vi "Rapid Filter Tester.vi"() -> ()   [LabVIEW 2012]
doc: "Changed serial pause logic for sending commands to the STAMP box to ensure that it can never be less than the minimum value.\n\nIncreased serial pause from 50 to 75 ms."
uses:
  file action.ctl
  Pump calibration/calibration commands.ctl
  Sample commands.ctl
  sample references.ctl
  Peristaltic/3-stop colors.ctl
  State Setting.ctl
  tanks.ctl
  tank.ctl
  Method settings.ctl
  column flow.ctl
  point.ctl
  vial position.ctl
  sampler states.ctl
  sample array.ctl
  legend.ctl
  toolbar icons/help.ctl
  Peristaltic/Pump.ctl
  mini peristaltic pump.ctl
  Pump Direction.ctl
  RACE  compact controls.ctl
  Stamp/Switch settings vertical.ctl
  flow fraction.ctl
panel:
  in  "Tab Control":enum32{"Method", "States", "Samples", "Run"}(tab)
  in  "Method settings":T1 {"Column"."porosity" format="%.4f"; "Column"."diameter" format="%.2f"; "Column"."length" format="%.2f"}
  in  "Test list":i32(listbox)
  in  "add cycle before":bool
  in  "delete cycle":bool
  in  "Test name":string="first cycle"
  in  "add cycle after":bool
  in  "State Settings":T3[][](array[typedef])=[[{"switches"={"Pump"=FALSE, "1"=FALSE, "2"=FALSE, "3"=FALSE, "4"=FALSE, "5"=FALSE, "6"=FALSE}, "flow rate"=0.0, "flow division"={"1"=0.0, "2"=0.0, "3"=0.0, "4"=0.0, "5"=0.0}, "State name"="", "state duration"=0.0, "valve cycle time"=0.2}]] {"valve cycle time" min=0.2 step=0.1 format="%.2f"; "flow division"."5" min=0.0 max=1.0 step=0.01 format="%.3f"; "flow division"."4" min=0.0 max=1.0 step=0.01 format="%.3f"; "flow division"."3" min=0.0 max=1.0 step=0.01 format="%.3f"; "flow division"."2" min=0.0 max=1.0 step=0.01 format="%.3f"; "flow division"."1" min=0.0 max=1.0 step=0.01 format="%.3f"; "flow rate" format="%.3f"}
  in  "Influent list":i32(listbox)
  in  "add state before":bool
  in  "delete state":bool
  in  "State name":string="first reagent"
  in  "add state after":bool
  out "Legend":T6
  in  "Sample array":T7 {"Sample volume" format="%.2f"; "Influent list" items=["first reagent"]; "Test list" items=["first cycle"]; "t/theta" min=0.0 step=0.1}
  in  "Index":i32
  in  "Plant Mode of Operation":T8(ring)=enum."Automatic Operation"
  in  "stop run":bool
  in  "Run":bool
  out "valve cycle time":dbl[unit] format="%.2f"
  in  "Help Button":T9
  in  "Calibrate Pump":T10 {"flow rate" format="%.2f"}
  out "Sample Tray":T12
  out "Sample plot":picture
  out "sampler state":T13
  out "vial position":T14
  out "run done":bool
  out "current time":dbl[unit]
  out "column flow":T15 {"t/q" format="%.3f"; "Velocity" format="%.3f"}
  in  "Which volumes":T16(ring)
  out "total run time":dbl[unit]
  out "update gui":bool=TRUE
  out "Elapsed time in current state":dbl[unit] format="%<%H:%M:%S%2u>t"
  in  "Reagents":string[](array[string])
  in  "New State":T3={"switches"={"Pump"=FALSE, "1"=FALSE, "2"=FALSE, "3"=FALSE, "4"=FALSE, "5"=FALSE, "6"=FALSE}, "flow rate"=0.0, "flow division"={"1"=0.0, "2"=0.0, "3"=0.0, "4"=0.0, "5"=0.0}, "State name"="", "state duration"=0.0, "valve cycle time"=0.2} {"valve cycle time" min=0.2 step=0.1 format="%.2f"; "flow division"."5" min=0.0 max=1.0 step=0.01 format="%.3f"; "flow division"."4" min=0.0 max=1.0 step=0.01 format="%.3f"; "flow division"."3" min=0.0 max=1.0 step=0.01 format="%.3f"; "flow division"."2" min=0.0 max=1.0 step=0.01 format="%.3f"; "flow division"."1" min=0.0 max=1.0 step=0.01 format="%.3f"; "flow rate" format="%.3f"}
  out "Quit":bool
  out "Control Settings":T17
  out "tanks":T20 {"Tank 5" scale format="%.1f"; "Tank 4" scale format="%.1f"; "Tank 3" scale format="%.1f"; "Tank 2" scale format="%.1f"; "Tank 1" scale format="%.1f"}
  # "sampler"
  # "waste"
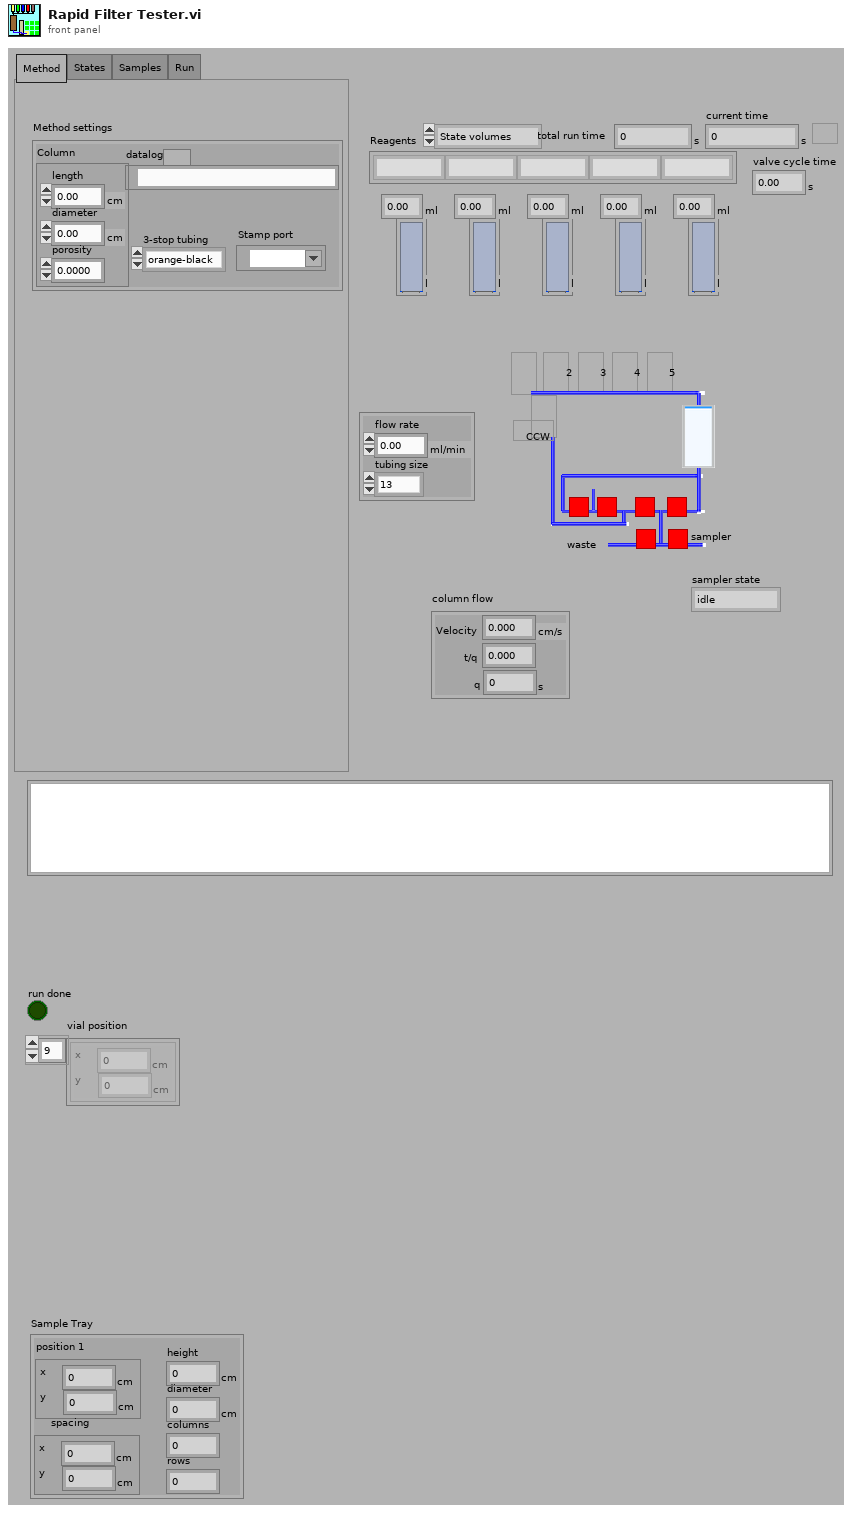
[diagram p1: front panel]
types:
  T1 = typedef "Method settings.ctl" = cluster{"3-stop tubing":T2, "Stamp port":refnum<visa-resource-name>, "datalog":path, "Column":cluster{"length":dbl[unit], "diameter":dbl[unit], "porosity":dbl}}
  T2 = typedef "3-stop colors.ctl" = enum16{"orange-black", "orange-red", "orange-blue", "orange-green", "green-yellow", "orange-yellow", "white-yellow", "orange-white", "black-black", "orange-orange", "white-black", "white-white", "white-red", "red-red", "red-grey", "grey-grey", "yellow-yellow", "yellow-blue", "blue-blue", "blue-green", "green-green", "purple-purple", "purple-black", "purple-orange", "purple-white", "black-white", "13", "14", "15", "16", "17", "18"}
  T3 = typedef "State Setting.ctl" = cluster{"switches":T4, "flow rate":dbl[unit], "flow division":cluster{"1":T5, "2":T5, "3":T5, "4":T5, "5":T5}, "State name":string, "state duration":dbl[unit], "valve cycle time":dbl[unit]}
  T4 = typedef "Switch settings vertical.ctl" = cluster{"Pump":bool, "1":bool, "2":bool, "3":bool, "4":bool, "5":bool, "6":bool}
  T5 = typedef "flow fraction.ctl" = dbl
  T6 = typedef "legend.ctl" = cluster{"Feed ":string, "Color":u32}[]
  T7 = typedef "sample array.ctl" = cluster{"start time":dbl[unit], "end time":dbl[unit], "t/theta":dbl, "Test list":u16, "Influent list":u16, "Sample volume":dbl[unit], "Too close to previous sample":bool}[]
  T8 = enum16{"Operator Selected State", "Automatic Operation"}
  T9 = typedef "help.ctl" = bool
  T10 = typedef "Pump.ctl" = cluster{"tubing size":enum16{"13", "14", "16", "25", "17", "18"}, "flow rate":dbl[unit]}
  T11 = typedef "point.ctl" = cluster{"x":dbl[unit], "y":dbl[unit]}
  T12 = cluster{"diameter":dbl[unit], "height":dbl[unit], "columns":u16, "rows":u16, "position 1":T11, "spacing":T11}
  T13 = typedef "sampler states.ctl" = enum16{"idle", "go sample loc", "collect sample", "go home"}
  T14 = typedef "vial position.ctl" = T11[]
  T15 = typedef "column flow.ctl" = cluster{"Velocity":dbl[unit], "t/q":dbl, "q":dbl[unit]}
  T16 = enum16{"State volumes", "Cycle volumes", "Experiment volumes"}
  T17 = typedef "RACE  compact controls.ctl" = cluster{"Switches":cluster{"1":T18, "2":T18, "3":T18, "4":T18, "5":T18, "Boolean":bool, "Boolean 2":bool, "Boolean 3":bool, "Boolean 4":bool, "Boolean 5":bool, "Boolean 6":bool, "main pump":T18, "direction":T19}}
  T18 = typedef "mini peristaltic pump.ctl" = bool
  T19 = typedef "Pump Direction.ctl" = bool
  T20 = typedef "tanks.ctl" = cluster{"Tank 1":T21, "Tank 2":T21, "Tank 3":T21, "Tank 4":T21, "Tank 5":T21}
  T21 = typedef "tank.ctl" = dbl[unit]
  T22 = typedef "calibration commands.ctl" = enum16{"Get ini Path", "Save default values", "Save new calibration", "Read calibration", "Apply calibration", "Read STAMP mb", "Write STAMP mb"}
  T23 = typedef "sample references.ctl" = cluster{"Index":refnum<vi>, "Test list":refnum<vi>, "Influent list":refnum<vi>, " State Settings":refnum<vi>, "Method settings":refnum<vi>, "Sample plot":refnum<vi>, "Legend":refnum<vi>, "Test Ring":refnum<vi>, "Influent Ring":refnum<vi>, "TabCtl Refnum":refnum<vi>, "Sample array":refnum<vi>}
  T24 = typedef "Sample commands.ctl" = enum16{"Configure", "Update times", "Index", "Update rings", "Plot current time"}
  T25 = typedef "file action.ctl" = enum16{"Save", "Open"}
  T26 = typedef "calibration values.ctl" = cluster{"target 1":dbl[unit], "target 2":dbl[unit], "measured 1":dbl[unit], "measured 2":dbl[unit]}
  T27 = typedef "Stamp Controls.ctl" = cluster{"Pump speed":dbl, "switches":T28}
  T28 = typedef "switches.ctl" = cluster{"Pump":bool, "1":bool, "2":bool, "3":bool, "4":bool, "5":bool, "6":bool}
  T29 = cluster{"Item Names":string[], "Value":i32, "Item Names":string[], "Value":i32, " State Settings":T3[][], "Method settings":T1, "Reagents":string[], "vial position":T14, "Sample array":T7, "Sample Tray":cluster{"diameter":dbl[unit], "height":dbl[unit], "columns":u16, "rows":u16, "position 1":T11, "spacing":T11}}
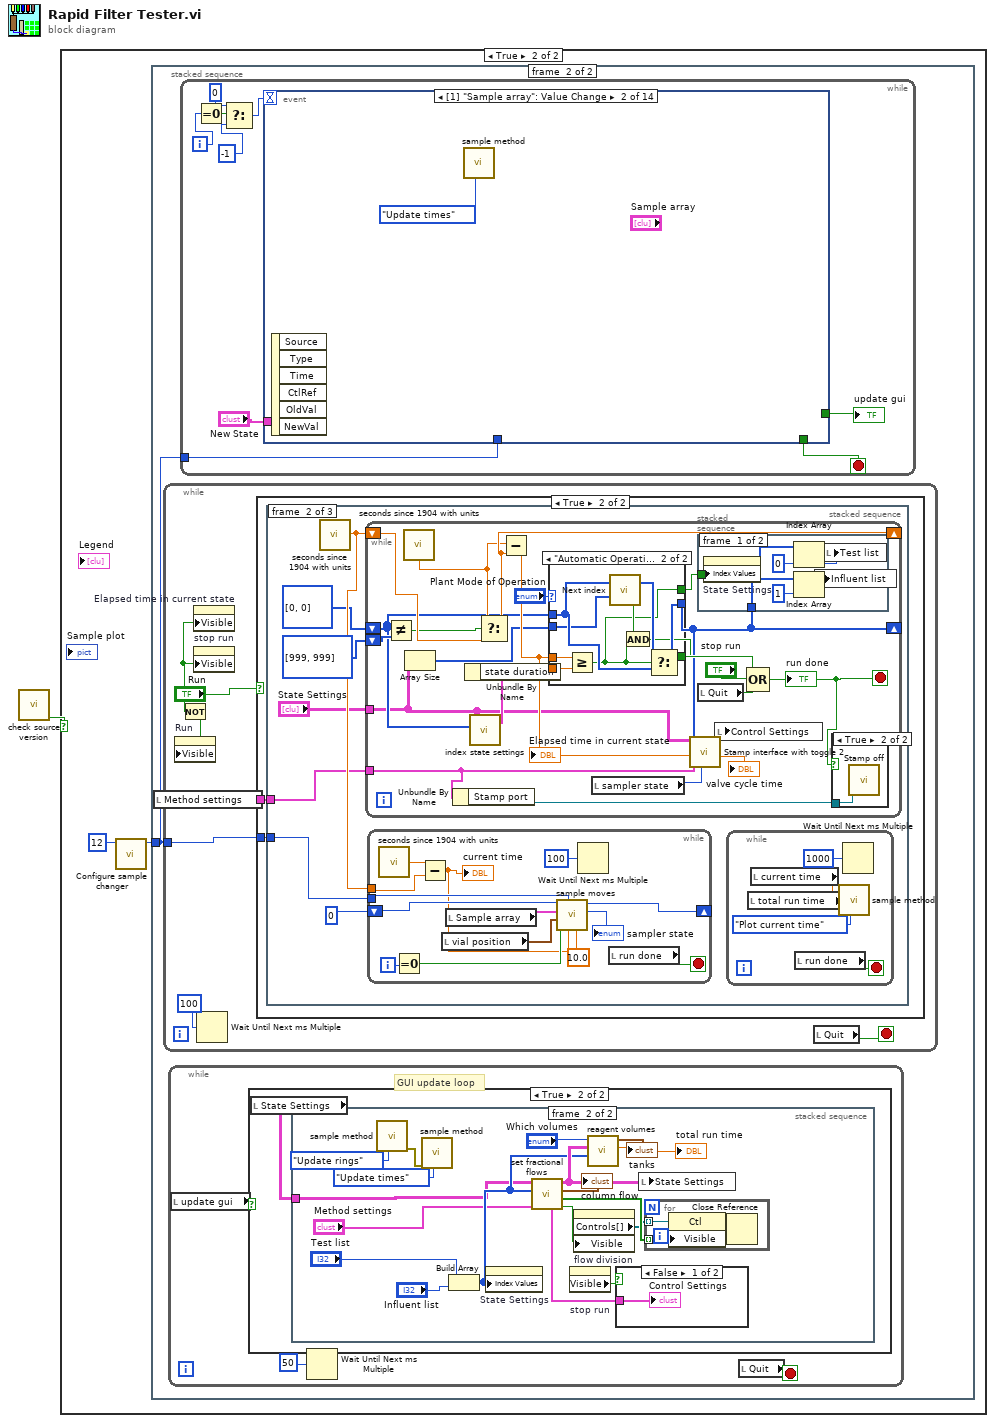
[diagram p0: block diagram]
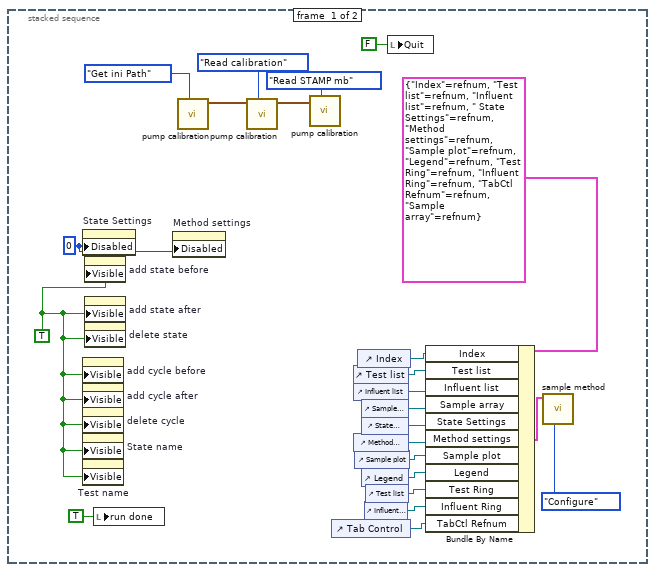
[diagram p3: hidden frame]
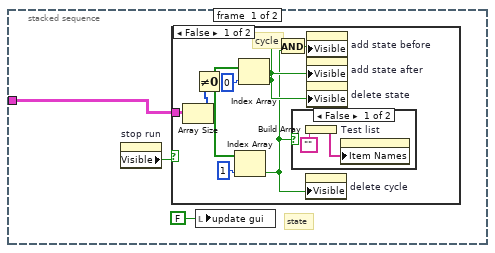
[diagram p5: hidden frame]
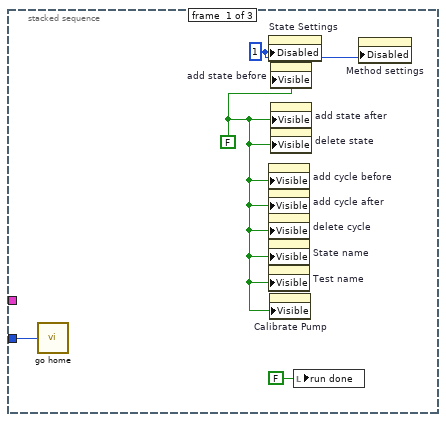
[diagram p10: hidden frame]
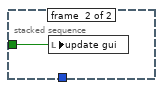
[diagram p12: hidden frame]
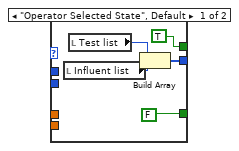
[diagram p13: hidden frame]
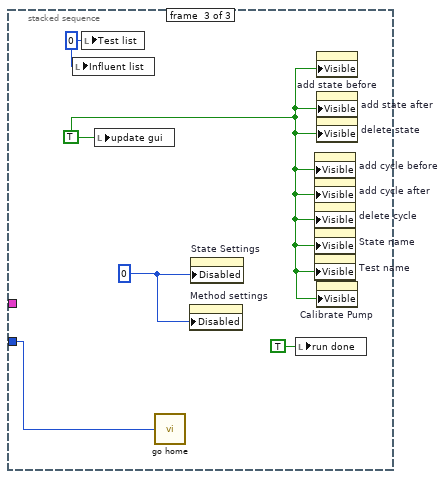
[diagram p14: hidden frame]
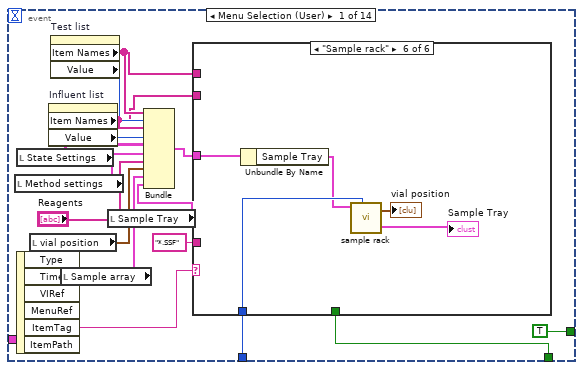
[diagram p15: hidden frame]
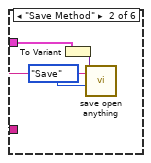
[diagram p17: hidden frame]
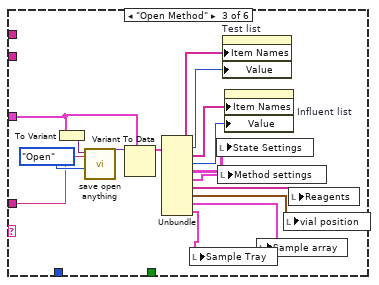
[diagram p18: hidden frame]
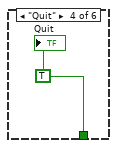
[diagram p19: hidden frame]
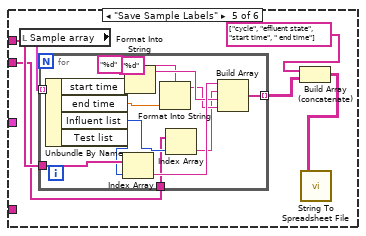
[diagram p20: hidden frame]
diagram:
  n1 = call "check source version.vi"() -> ("continue running?"=w1:bool)  [unwired: 2 in, 3 out]
  n2 = case shown="True" w1 {
    frame False {
    }
    frame True {
      n3 = call "Configure sample changer.vi"("ID"=12) -> ("ID out"=w2:i32)  [unwired: 6 in]
      n4 = stacked-sequence {
        tunnel: w2 -> [_ w27]
        frame #0 {
          w24 = u8 0 ("Disabled")
          w25 = TRUE
          n5 = property on="State Settings" class="Arr (strict)"("Disabled"=w24) -> ()  [unwired: 2 in, 2 out]
          n6 = property on="add cycle before" class="Bool"("Visible"=w25) -> ()  [unwired: 2 in, 2 out]
          n7 = property on="add cycle after" class="Bool"("Visible"=w25) -> ()  [unwired: 2 in, 2 out]
          n8 = property on="delete cycle" class="Bool"("Visible"=w25) -> ()  [unwired: 2 in, 2 out]
          n9 = property on="State name" class="Str"("Visible"=w25) -> ()  [unwired: 2 in, 2 out]
          n10 = property on="Test name" class="Str"("Visible"=w25) -> ()  [unwired: 2 in, 2 out]
          n11 = property on="add state before" class="Bool"("Visible"=w25) -> ()  [unwired: 2 in, 2 out]
          n12 = property on="add state after" class="Bool"("Visible"=w25) -> ()  [unwired: 2 in, 2 out]
          n13 = property on="delete state" class="Bool"("Visible"=w25) -> ()  [unwired: 2 in, 2 out]
          n14 = local write "run done"(TRUE ("run done")) -> ()
          n15 = property on="Method settings" class="Clust (strict)"("Disabled"=w24) -> ()  [unwired: 2 in, 2 out]
          n16 = call "pump calibration.vi"("pump cal command"=calibration_commands."Get ini Path") -> ("Pump Calibration out"=w21:T26)  [unwired: 4 in, 3 out]
          n17 = call "pump calibration.vi"("pump cal command"=calibration_commands."Read calibration", "Pump Calibration in"=w21) -> ("Pump Calibration out"=w5:T26)  [unwired: 3 in, 3 out]
          n18 = call "pump calibration.vi"("pump cal command"=calibration_commands."Read STAMP mb", "Pump Calibration in"=w5) -> ()  [unwired: 3 in, 4 out]
          n19 = control-ref of="Tab Control"() -> (w7:refnum<vi>)
          n20 = control-ref of="Test list"() -> (w16:refnum<vi>)
          n21 = control-ref of="Influent list"() -> (w15:refnum<vi>)
          n22 = control-ref of="Method settings"() -> (w12:refnum<vi>)
          n23 = control-ref of="Sample plot"() -> (w11:refnum<vi>)
          n24 = control-ref of="Index"() -> (w17:refnum<vi>)
          n25 = control-ref of="Sample array"() -> (w14:refnum<vi>)
          n26 = control-ref of="State Settings"() -> (w13:refnum<vi>)
          n27 = control-ref of="Legend"() -> (w10:refnum<vi>)
          n28 = control-ref of="Influent list"() -> (w8:refnum<vi>)
          n29 = control-ref of="Test list"() -> (w9:refnum<vi>)
          n30 = local write "Quit"(FALSE ("Quit")) -> ()
          n31 = Bundle By Name(cluster=T23 {"Index"=refnum, "Test list"=refnum, "Influent list"=refnum, " State Settings"=refnum, "Method settings"=refnum, "Sample plot"=refnum, "Legend"=refnum, "Test Ring"=refnum, "Influent Ring"=refnum, "TabCtl Refnum"=refnum, "Sample array"=refnum} ("Ref cluster"), "Index"=w17, "Test list"=w16, "Influent list"=w15, "Sample array"=w14, "State Settings"=w13, "Method settings"=w12, "Sample plot"=w11, "Legend"=w10, "Test Ring"=w9, "Influent Ring"=w8, "TabCtl Refnum"=w7) -> (w18:T23)
          n32 = call "sample method.vi"("Sample Commands"=Sample_commands."Configure", "Ref cluster"=w18) -> ()  [unwired: 9 in, 1 out]
        }
        frame #1 {
          n33 = while {
            tunnel: w27 -> [w69]
            stop <- w71 stop-if-true
            n34 = local read "Method settings"() -> (w68:T1)
            n35 = Not(x="Run") -> (.not. x?=w72:bool)
            n36 = property on="Run" class="Bool"("Visible"=w72) -> ()  [unwired: 2 in, 2 out]
            n37 = property on="Elapsed time in current state" class="DigNum (strict)"("Visible"="Run") -> ()  [unwired: 2 in, 2 out]
            n38 = property on="stop run" class="Bool"("Visible"="Run") -> ()  [unwired: 2 in, 2 out]
            n39 = Wait Until Next ms Multiple(millisecond multiple=u32 100) -> ()  [unwired: 1 out]
            n40 = case shown="True" "Run" {
              tunnel: w69 -> [_ w74]
              tunnel: w68 -> [_ w73]
              frame False {
              }
              frame True {
                n41 = stacked-sequence {
                  tunnel: w74 -> [w76 w82 w150]
                  tunnel: w73 -> [_ w79 _]
                  frame #0 {
                    w77 = u8 1 ("Disabled")
                    w75 = FALSE
                    n42 = call "go home.vi"("ID in"=w76) -> ()
                    n43 = property on="State Settings" class="Arr (strict)"("Disabled"=w77) -> ()  [unwired: 2 in, 2 out]
                    n44 = property on="add cycle before" class="Bool"("Visible"=w75) -> ()  [unwired: 2 in, 2 out]
                    n45 = property on="add cycle after" class="Bool"("Visible"=w75) -> ()  [unwired: 2 in, 2 out]
                    n46 = property on="delete cycle" class="Bool"("Visible"=w75) -> ()  [unwired: 2 in, 2 out]
                    n47 = property on="State name" class="Str"("Visible"=w75) -> ()  [unwired: 2 in, 2 out]
                    n48 = property on="Test name" class="Str"("Visible"=w75) -> ()  [unwired: 2 in, 2 out]
                    n49 = property on="Calibrate Pump" class="Clust (strict)"("Visible"=w75) -> ()  [unwired: 2 in, 2 out]
                    n50 = property on="add state before" class="Bool"("Visible"=w75) -> ()  [unwired: 2 in, 2 out]
                    n51 = property on="add state after" class="Bool"("Visible"=w75) -> ()  [unwired: 2 in, 2 out]
                    n52 = property on="delete state" class="Bool"("Visible"=w75) -> ()  [unwired: 2 in, 2 out]
                    n53 = local write "run done"(FALSE ("run done")) -> ()
                    n54 = property on="Method settings" class="Clust (strict)"("Disabled"=w77) -> ()  [unwired: 2 in, 2 out]
                  }
                  frame #1 {
                    n55 = call "seconds since 1904 with units.vi"() -> ("seconds since 1Jan1904"=w84:dbl[unit])
                    n56 = while {
                      shift-right: [w115] -> _
                      shift-left: u32[] [999, 999] ("Index Values") -> [w122]
                      shift-left: u32[] [0, 0] ("Index Values") -> [w109]
                      shift-right: [w125] -> _
                      shift-left: w84 -> [w126]
                      tunnel: "State Settings" -> [w108]
                      tunnel: w79 -> [w106]
                      stop <- w105 stop-if-true
                      n57 = Not Equal?(x=w109, y=w122) -> (x != y?=w114:bool)
                      n58 = call "seconds since 1904 with units.vi"() -> ("seconds since 1Jan1904"=w112:dbl[unit])
                      n59 = Array Size(array=w108) -> (size(s)=w116:i32[])
                      n60 = Unbundle By Name(w106) -> ("Stamp port"=w107:refnum<visa-resource-name>)
                      n61 = call "index state settings.vi"("Next Index"=w109, "State Settings"=w108) -> ("State"=w118:T3)  [unwired: 2 in, 1 out]
                      n62 = Unbundle By Name(w118) -> ("state duration"=w124:dbl[unit])
                      n63 = Select(t=w112, s=w114, f=w126) -> (s? t:f=w125:dbl[unit])
                      n64 = Subtract(x=w112, y=w125) -> (x-y=w123:dbl[unit])
                      "Elapsed time in current state" <- w123
                      n65 = case shown="\"Automatic Operation\"" "Plant Mode of Operation" {
                        tunnel: [w137 w145] -> w115
                        tunnel: w123 -> [_ w148]
                        tunnel: w124 -> [_ w147]
                        tunnel: w109 -> [_ w144]
                        tunnel: [FALSE ("last state") w141] -> w119
                        tunnel: w116 -> [_ w143]
                        tunnel: [TRUE w140] -> w113
                        frame "Operator Selected State", Default {
                          n66 = local read "Influent list"() -> (w138:i32)
                          n67 = local read "Test list"() -> (w139:i32)
                          n68 = Build Array(w139, w138) -> (w137:i32[])
                        }
                        frame "Automatic Operation" {
                          n69 = Greater Or Equal?(x=w148, y=w147) -> (x >= y?=w140:bool)
                          n70 = call "Next index.vi"("size(s)"=w143, "Current Index"=w144) -> ("last state"=w142:bool, "Next Index"=w146:u32[])
                          n71 = And(x=w142, y=w140) -> (x .and. y?=w141:bool)
                          n72 = Select(t=w146, s=w140, f=w144) -> (s? t:f=w145:u32[])
                        }
                      }
                      n73 = local read "sampler state"() -> (w111:T13)
                      n74 = call "Stamp interface with toggle 2.vi"("sampler state"=w111, "Elapsed time in current state"=w123, "Method settings"=w106, "Index"=w115, "State Settings"=w108) -> ("valve cycle time"=→"valve cycle time":dbl[unit], "Controls out"=w117:T27)  [unwired: 4 in, 1 out]
                      n75 = stacked-sequence {
                        tunnel: w115 -> [w132 _]
                        tunnel: w113 -> [_ w134]
                        frame #0 {
                          n76 = property on="State Settings" class="Arr (strict)"("Index Values"=w132) -> ()  [unwired: 2 in, 2 out]
                          n77 = Index Array(array=w132, index=0) -> (element=w133:u32)
                          n78 = Index Array(array=w132, index=1) -> (element=w131:u32)
                          n79 = local write "Influent list"(w131) -> ()
                          n80 = local write "Test list"(w133) -> ()
                        }
                        frame #1 {
                          n81 = local write "update gui"(w134) -> ()
                        }
                      }
                      n82 = local read "Quit"() -> (w120:bool)
                      n83 = local write "Control Settings"(w117) -> ()
                      n84 = Compound Arithmetic op=OR(w119, "stop run", w120) -> (w105:bool)
                      "run done" <- w105
                      n85 = case shown="True" w105 {
                        tunnel: w107 -> [_ w128]
                        frame False {
                        }
                        frame True {
                          n86 = call "Stamp off.vi"("Serial Port"=w128) -> ()  [unwired: 9 in, 2 out]
                        }
                      }
                    }
                    n87 = while {
                      tunnel: w84 -> [w102]
                      shift-right: [w100] -> _
                      shift-left: 0 -> [w101]
                      tunnel: w82 -> [w97]
                      i -> [w93]
                      stop <- w104 stop-if-true
                      n88 = call "seconds since 1904 with units.vi"() -> ("seconds since 1Jan1904"=w103:dbl[unit])
                      n89 = Equal To 0?(x=w93) -> (x = 0?=w92:bool)
                      n90 = Subtract(x=w103, y=w102) -> (x-y=w91:dbl[unit])
                      "current time" <- w91
                      n91 = local read "vial position"() -> (w94:T14)
                      n92 = local read "Sample array"() -> (w98:T7)
                      n93 = call "sample moves.vi"("move time"=dbl[unit] 10.0, "current time"=w91, "Gilson ID"=w97, "initialize"=w92, "vial position"=w94, "Samples"=w98, "sample ID"=w101) -> ("sampler state"=→"sampler state":T13, "sample ID out"=w100:i16)  [unwired: 3 in]
                      n94 = Wait Until Next ms Multiple(millisecond multiple=u32 100) -> ()  [unwired: 1 out]
                      n95 = local read "run done"() -> (w104:bool)
                    }
                    n96 = while {
                      stop <- w90 stop-if-true
                      n97 = local read "total run time"() -> (w88:dbl[unit])
                      n98 = local read "current time"() -> (w87:dbl[unit])
                      n99 = local read "run done"() -> (w90:bool)
                      n100 = call "sample method.vi"("Sample Commands"=Sample_commands."Plot current time", "total run time"=w88, "current time"=w87) -> ()  [unwired: 8 in, 1 out]
                      n101 = Wait Until Next ms Multiple(millisecond multiple=u32 1000) -> ()  [unwired: 1 out]
                    }
                  }
                  frame #2 {
                    w151 = u8 0 ("Disabled")
                    w153 = 0 ("Cycle list")
                    w149 = TRUE ("update gui")
                    n102 = local write "Influent list"(w153) -> ()
                    n103 = local write "Test list"(w153) -> ()
                    n104 = local write "update gui"(w149) -> ()
                    n105 = call "go home.vi"("ID in"=w150) -> ()
                    n106 = property on="Method settings" class="Clust (strict)"("Disabled"=w151) -> ()  [unwired: 2 in, 2 out]
                    n107 = property on="State Settings" class="Arr (strict)"("Disabled"=w151) -> ()  [unwired: 2 in, 2 out]
                    n108 = local write "run done"(TRUE ("run done")) -> ()
                    n109 = property on="add cycle before" class="Bool"("Visible"=w149) -> ()  [unwired: 2 in, 2 out]
                    n110 = property on="add cycle after" class="Bool"("Visible"=w149) -> ()  [unwired: 2 in, 2 out]
                    n111 = property on="delete cycle" class="Bool"("Visible"=w149) -> ()  [unwired: 2 in, 2 out]
                    n112 = property on="State name" class="Str"("Visible"=w149) -> ()  [unwired: 2 in, 2 out]
                    n113 = property on="Test name" class="Str"("Visible"=w149) -> ()  [unwired: 2 in, 2 out]
                    n114 = property on="add state before" class="Bool"("Visible"=w149) -> ()  [unwired: 2 in, 2 out]
                    n115 = property on="add state after" class="Bool"("Visible"=w149) -> ()  [unwired: 2 in, 2 out]
                    n116 = property on="delete state" class="Bool"("Visible"=w149) -> ()  [unwired: 2 in, 2 out]
                    n117 = property on="Calibrate Pump" class="Clust (strict)"("Visible"=w149) -> ()  [unwired: 2 in, 2 out]
                  }
                }
              }
            }
            n118 = local read "Quit"() -> (w71:bool)
          }
          n119 = while {
            stop <- w29 stop-if-true
            # "GUI update loop"
            n120 = local read "update gui"() -> (w28:bool)
            n121 = case shown="True" w28 {
              frame False {
              }
              frame True {
                n122 = local read "State Settings"() -> (w31:T3[][])
                n123 = stacked-sequence {
                  tunnel: w31 -> [w34 w48]
                  frame #0 {
                    # "state"
                    n124 = property on="stop run" class="Bool"() -> ("Visible"=w32:bool)  [unwired: 2 in, 2 out]
                    n125 = case shown="False" w32 {
                      tunnel: w34 -> [w36 _]
                      frame False {
                        # "cycle"
                        n126 = Array Size(array=w36) -> (size(s)=w39:i32[])
                        n127 = Not Equal To 0?(x=w39) -> (x != 0?=w40:bool[])
                        n128 = Index Array(array=w40, index=1) -> (element=w35:bool)
                        n129 = Index Array(array=w40, index=0) -> (element=w41:bool)
                        n130 = And(x=w41, y=w35) -> (x .and. y?=w42:bool)
                        n131 = case shown="False" w35 {
                          frame False {
                            n132 = Build Array("") -> (w43:string[])
                            n133 = property on="Test list" class="LstBox (strict)"("Item Names"=w43) -> ()  [unwired: 2 in, 2 out]
                          }
                          frame True {
                          }
                        }
                        n134 = property on="delete cycle" class="Bool"("Visible"=w35) -> ()  [unwired: 2 in, 2 out]
                        n135 = property on="add state before" class="Bool"("Visible"=w42) -> ()  [unwired: 2 in, 2 out]
                        n136 = property on="add state after" class="Bool"("Visible"=w41) -> ()  [unwired: 2 in, 2 out]
                        n137 = property on="delete state" class="Bool"("Visible"=w41) -> ()  [unwired: 2 in, 2 out]
                      }
                      frame True {
                      }
                    }
                    n138 = local write "update gui"(FALSE ("update gui")) -> ()
                  }
                  frame #1 {
                    n139 = call "sample method.vi"("Sample Commands"=Sample_commands."Update rings") -> ("error out"=w45:errorcluster)  [unwired: 10 in]
                    n140 = call "sample method.vi"("Sample Commands"=Sample_commands."Update times", "error in (no error)"=w45) -> ()  [unwired: 9 in, 1 out]
                    n141 = Build Array("Test list", "Influent list") -> (w54:i32[])
                    n142 = property on="State Settings" class="Arr (strict)"("Index Values"=w54) -> ()  [unwired: 2 in, 2 out]
                    n143 = call "set fractional flows.vi"("State Settings"=w48, "Index Values"=w54, "Method settings"="Method settings") -> ("Control Settings"=w60:T27, "State Settings out"=w61:T3[][], "column flow"=→"column flow":T15, "toggle valves"=w58:bool[], "show fractions"=w59:bool)  [unwired: 2 in]
                    n144 = property on="stop run" class="Bool"() -> ("Visible"=w56:bool)  [unwired: 2 in, 2 out]
                    n145 = property on="flow division" class="Clust (strict)"("Visible"=w59) -> ("Controls[]"=w57:refnum<vi>[])  [unwired: 2 in, 2 out]
                    n146 = call "reagent volumes.vi"("Index Values"=w54, "State Settings"=w61, "Which volumes"="Which volumes") -> ("total run time"=→"total run time":dbl[unit], "tanks"=→"tanks":T20)  [unwired: 7 in]
                    n147 = case shown="False" w56 {
                      tunnel: w60 -> [w63 _]
                      frame False {
                        "Control Settings" <- w63
                      }
                      frame True {
                      }
                    }
                    n148 = local write "State Settings"(w61) -> ()
                    n149 = for {
                      tunnel: w57 -> [w66] mode=indexing
                      tunnel: w58 -> [w65] mode=indexing
                      n150 = property class="Ctl"(reference=w66, "Visible"=w65) -> (reference out=w64:refnum<vi>)  [unwired: 1 in, 1 out]
                      n151 = Close Reference(reference=w64) -> ()  [unwired: 1 in, 1 out]
                    }
                  }
                }
              }
            }
            n152 = Wait Until Next ms Multiple(millisecond multiple=u32 50) -> ()  [unwired: 1 out]
            n153 = local read "Quit"() -> (w29:bool)
          }
          n154 = while {
            tunnel: w27 -> [w154]
            i -> [w158]
            stop <- w162 stop-if-true
            n155 = Equal To 0?(x=w158) -> (x = 0?=w159:bool)
            n156 = Select(t=0, s=w159, f=-1) -> (s? t:f=w155:i32)
            n157 = event shown="[1] \"Sample array\": Value Change" {
              selector: _ -> [_ _ _ _ _ _ _ _ _ _ _ _ _ _]
              dyn-events: _ -> [_ _ _ _ _ _ _ _ _ _ _ _ _ _]
              timeout: w155 -> [_ _ _ _ _ _ _ _ _ _ _ _ _ _]
              tunnel: [w177 _ _ _ _ w238 _ _ _ _ _ _ _ _] -> w162
              tunnel: "New State" -> [_ _ _ _ _ _ w244 w285 _ _ _ _ _ _]
              tunnel: [TRUE ("update gui") _ _ _ TRUE ("update gui") _ TRUE ("update gui") TRUE ("update gui") TRUE ("update gui") TRUE ("update gui") _ TRUE ("update gui") TRUE ("update gui") TRUE ("update gui")] -> w160
              tunnel: w154 -> [w167 _ _ _ _ _ _ _ _ _ _ _ _ _]
              event Menu Selection (User) {
                n158 = local read "Method settings"() -> (w174:T1)
                n159 = local read "State Settings"() -> (w172:T3[][])
                n160 = event-data() -> ("ItemTag"=w178:string)  [unwired: 1 in, 5 out]
                n161 = local read "vial position"() -> (w166:T14)
                n162 = property on="Influent list" class="LstBox (strict)"() -> ("Item Names"=w163:string[], "Value"=w170:i32)  [unwired: 2 in, 2 out]
                n163 = property on="Test list" class="LstBox (strict)"() -> ("Item Names"=w169:string[], "Value"=w171:i32)  [unwired: 2 in, 2 out]
                n164 = local read "Sample array"() -> (w165:T7)
                n165 = local read "Sample Tray"() -> (w164:T12)
                n166 = Bundle("Item Names"=w169, "Value"=w171, "Item Names"=w163, "Value"=w170, "State Settings"=w172, "Method settings"=w174, "Reagents"="Reagents", "vial position"=w166, "Sample array"=w165, "Sample Tray"=w164) -> (w175:T29)  [unwired: 1 in]
                n167 = case shown="\"Sample rack\"" w178 {
                  tunnel: [_ _ _ w199 _ _] -> w177
                  tunnel: "*.SSF" ("pattern") -> [_ w181 w197 _ _ _]
                  tunnel: w175 -> [_ w179 w195 _ _ w222]
                  tunnel: w169 -> [_ _ _ _ w204 _]
                  tunnel: w167 -> [_ _ _ _ _ w223]
                  tunnel: w163 -> [_ _ _ _ w200 _]
                  frame "False", Default {
                  }
                  frame "Save Method" {
                    n168 = To Variant(anything=w179) -> (Variant=w180:variant)
                    n169 = call "save open anything.vi"("Variant"=w180, "Action"=file_action."Save", "pattern"=w181) -> ()  [unwired: 4 in, 4 out]
                  }
                  frame "Open Method" {
                    n170 = To Variant(anything=w195) -> (Variant=w194:variant)
                    n171 = call "save open anything.vi"("Variant"=w194, "Action"=file_action."Open", "pattern"=w197) -> ("Variant out"=w196:variant)  [unwired: 4 in, 3 out]
                    n172 = Variant To Data(type=w195, Variant=w196) -> (data=w193:T29)  [unwired: 1 in, 1 out]
                    n173 = Unbundle(w193) -> ("Item Names"=w187:string[], "Value"=w189:i32, "Item Names"=w186:string[], "Value"=w188:i32, "State Settings"=w190:T3[][], "Method settings"=w191:T1, "Reagents"=w192:string[], "vial position"=w185:T14, "Sample array"=w184:T7, "Sample Tray"=w183:T12)
                    n174 = local write "Sample Tray"(w183) -> ()
                    n175 = local write "State Settings"(w190) -> ()
                    n176 = local write "Method settings"(w191) -> ()
                    n177 = property on="Test list" class="LstBox (strict)"("Item Names"=w187, "Value"=w189) -> ()  [unwired: 2 in, 2 out]
                    n178 = property on="Influent list" class="LstBox (strict)"("Item Names"=w186, "Value"=w188) -> ()  [unwired: 2 in, 2 out]
                    n179 = local write "Sample array"(w184) -> ()
                    n180 = local write "vial position"(w185) -> ()
                    n181 = local write "Reagents"(w192) -> ()
                  }
                  frame "Quit" {
                    w199 = TRUE
                    "Quit" <- w199
                  }
                  frame "Save Sample Labels" {
                    n182 = local read "Sample array"() -> (w205:T7)
                    n183 = for {
                      tunnel: w205 -> [w219] mode=indexing
                      tunnel: w204 -> [w218]
                      tunnel: [w211] -> w202 mode=indexing
                      tunnel: w200 -> [w207]
                      n184 = Unbundle By Name(w219) -> ("start time"=w216:dbl[unit], "end time"=w215:dbl[unit], "Influent list"=w208:u16, "Test list"=w217:u16)
                      n185 = Index Array(array=w218, index=w217) -> (element=w214:string)
                      n186 = Format Into String(format string="%d", w216) -> (resulting string=w213:string)  [unwired: 2 in, 1 out]
                      n187 = Format Into String(format string="%d", w215) -> (resulting string=w212:string)  [unwired: 2 in, 1 out]
                      n188 = Index Array(array=w207, index=w208) -> (element=w206:string)
                      n189 = Build Array(w214, w206, w213, w212) -> (w211:string[])
                    }
                    n190 = Build Array (concatenate)(string[] ["cycle", "effluent state", "start time", " end time"] ("appended array"), w202) -> (w201:string[][])
                    n191 = call "String To Spreadsheet File.vi"("2D data"=w201) -> ()  [unwired: 7 in, 1 out]
                  }
                  frame "Sample rack" {
                    n192 = Unbundle By Name(w222) -> ("Sample Tray"=w221:T12)
                    n193 = call "sample rack.vi"("Sample Tray"=w221, "Gilson ID"=w223) -> ("vial position"=→"vial position":T14, "Sample Tray out"=→"Sample Tray":T12)  [unwired: 2 in, 1 out]
                  }
                }
              }
              event Value Change {
                n194 = event-data() -> ()  [unwired: 1 in, 6 out]
                n195 = call "sample method.vi"("Sample Commands"=Sample_commands."Update times") -> ()  [unwired: 10 in, 1 out]
              }
              event "Tab Control": Value Change {
                n196 = event-data() -> ("OldVal"=w226:enum32{"Method", "States", "Samples", "Run"})  [unwired: 1 in, 5 out]
                n197 = local read "run done"() -> (w229:bool)
                n198 = Equal?(x=enum32{"Method", "Samples", "Run"}."Run" ("Tab Control"), y=w226) -> (x = y?=w230:bool)
                n199 = Not(x=w229) -> (.not. x?=w228:bool)
                n200 = And(x=w228, y=w230) -> (x .and. y?=w227:bool)
                n201 = case shown="True" w227 {
                  tunnel: w226 -> [_ w233]
                  frame False {
                  }
                  frame True {
                    n202 = local write "Tab Control"(w233) -> ()
                  }
                }
                n203 = call "sample method.vi"("Sample Commands"=Sample_commands."Update times") -> ()  [unwired: 10 in, 1 out]
              }
              event "Index": Value Change {
                n204 = event-data() -> ()  [unwired: 1 in, 6 out]
                n205 = call "sample method.vi"("Sample Commands"=Sample_commands."Index") -> ("error out"=w234:errorcluster)  [unwired: 10 in]
                n206 = call "sample method.vi"("Sample Commands"=Sample_commands."Update times", "error in (no error)"=w234) -> ()  [unwired: 9 in, 1 out]
              }
              event Value Change {
                n207 = event-data() -> ()  [unwired: 1 in, 6 out]
                n208 = call "pump calibration dialog.vi"() -> ()  [unwired: 1 in]
              }
              event Panel Close {
                w238 = TRUE
                n209 = event-data() -> ()  [unwired: 1 in, 4 out]
                n210 = local write "Quit"(w238) -> ()
              }
              event "add cycle after", "add cycle before": Value Change {
                n211 = event-data() -> ()  [unwired: 1 in, 5 out]
                n212 = local read "State Settings"() -> (w251:T3[][])
                n213 = Array Size(array=w251) -> (size(s)=w248:i32[])
                n214 = Index Array(array=w248, index=1) -> (element=w246:i32)
                n215 = Equal To 0?(x=w246) -> (x = 0?=w245:bool)
                n216 = property on="Test list" class="LstBox (strict)"() -> ("Item Names"=w254:string[], "Value"=w253:i32)  [unwired: 2 in, 2 out]
                n217 = Increment(x=w253) -> (x+1=w252:i32)
                n218 = Select(t=w253, s="add cycle before", f=w252) -> (s? t:f=w240:i32)
                n219 = case shown="True" w245 {
                  tunnel: w253 -> [w262 _]
                  tunnel: w251 -> [w261 _]
                  tunnel: [w260 w270] -> w250
                  tunnel: w240 -> [w258 _]
                  tunnel: w244 -> [_ w265]
                  tunnel: "New cycle" ("Cycle name") -> [w257 w268]
                  tunnel: w254 -> [w256 _]
                  tunnel: [w255 w267] -> w239
                  frame False {
                    n220 = Index Array(array=w261, index (row)=w262) -> (element=w259:T3[])  [unwired: 1 in]
                    n221 = Insert Into Array(array=w256, index=w258, new element=w257) -> (w255:string[])
                    n222 = Insert Into Array(array=w261, index (row)=w258, new element=w259) -> (w260:T3[][])  [unwired: 1 in]
                  }
                  frame True {
                    w269 = 1 ("dimension size")
                    n223 = local read "State name"() -> (w264:string)
                    n224 = Bundle By Name(cluster=w265, "Influent name"=w264) -> (w266:T3)
                    n225 = Initialize Array(w268, w269) -> (w267:string[])
                    n226 = Build Array(w264) -> (w263:string[])
                    n227 = Initialize Array(w266, w269, w269) -> (w270:T3[][])
                    n228 = property on="Influent list" class="LstBox (strict)"("Item Names"=w263) -> ()  [unwired: 2 in, 2 out]
                  }
                }
                n229 = local write "State Settings"(w250) -> ()
                n230 = property on="Test list" class="LstBox (strict)"("Item Names"=w239, "Value"=w240) -> ()  [unwired: 2 in, 2 out]
                n231 = Index Array(array=w239, index=w240) -> (element=w241:string)
                n232 = local write "Test name"(w241) -> ()
              }
              event "add state after", "add state before": Value Change {
                w274 = "new reagent" ("State name")
                n233 = event-data() -> ()  [unwired: 1 in, 5 out]
                n234 = property on="Influent list" class="LstBox (strict)"() -> (error out=w286:errorcluster, "Item Names"=w277:string[], "Value"=w284:i32)  [unwired: 2 in, 1 out]
                n235 = local read "State Settings"() -> (w282:T3[][])
                n236 = Increment(x=w284) -> (x+1=w283:i32)
                n237 = Bundle By Name(cluster=w285, "Influent name"=w274) -> (w279:T3)
                n238 = Select(t=w284, s="add state before", f=w283) -> (s? t:f=w272:i32)
                n239 = Array Size(array=w277) -> (size(s)=w276:i32)
                n240 = Initialize Array(w279, w276) -> (w278:T3[])
                n241 = Insert Into Array(array=w277, index=w272, new element=w274) -> (w271:string[])
                n242 = Insert Into Array(array=w282, index (col)=w272, new element=w278) -> (w281:T3[][])  [unwired: 1 in]
                n243 = local write "State Settings"(w281) -> ()
                n244 = property on="Influent list" class="LstBox (strict)"(error in=w286, "Item Names"=w271, "Value"=w272) -> ()  [unwired: 1 in, 2 out]
                n245 = Index Array(array=w271, index=w272) -> (element=w273:string)
                n246 = local write "State name"(w273) -> ()
              }
              event "delete cycle": Value Change {
                n247 = event-data() -> ()  [unwired: 1 in, 5 out]
                n248 = property on="Test list" class="LstBox (strict)"() -> ("Item Names"=w292:string[], "Value"=w291:i32)  [unwired: 2 in, 2 out]
                n249 = local read "State Settings"() -> (w288:T3[][])
                n250 = Delete From Array(array=w292, length=1, index=w291) -> (array with subset deleted=w290:string[])  [unwired: 1 out]
                n251 = Delete From Array(array=w288, length=1, index (row)=w291) -> (array with subset deleted=w289:T3[][])  [unwired: 1 in, 1 out]
                n252 = property on="Test list" class="LstBox (strict)"("Item Names"=w290) -> ()  [unwired: 2 in, 2 out]
                n253 = local write "State Settings"(w289) -> ()
              }
              event "delete state": Value Change {
                n254 = event-data() -> ()  [unwired: 1 in, 5 out]
                n255 = property on="Influent list" class="LstBox (strict)"() -> ("Item Names"=w300:string[], "Value"=w296:i32)  [unwired: 2 in, 2 out]
                n256 = local read "State Settings"() -> (w297:T3[][])
                n257 = Delete From Array(array=w300, length=1, index=w296) -> (array with subset deleted=w299:string[])  [unwired: 1 out]
                n258 = Delete From Array(array=w297, length=1, index (col)=w296) -> (array with subset deleted=w298:T3[][])  [unwired: 1 in, 1 out]
                n259 = property on="Influent list" class="LstBox (strict)"("Item Names"=w299) -> ()  [unwired: 2 in, 2 out]
                n260 = local write "State Settings"(w298) -> ()
              }
              event Value Change {
                n261 = event-data() -> ()  [unwired: 1 in, 6 out]
                n262 = call "Web Browser.vi"("URL"="http://ceeserver.cee.cornell.edu/mw24/Software/Filter Tester.htm") -> ()  [unwired: 1 in]
              }
              event "State Settings", "Influent list", "Test list", "Which volumes": Value Change; Timeout {
                n263 = event-data() -> ()  [unwired: 1 in, 2 out]
                n264 = local read "Influent list"() -> (w305:i32)
                n265 = property on="Influent list" class="LstBox (strict)"() -> ("Item Names"=w304:string[])  [unwired: 2 in, 2 out]
                n266 = local read "Test list"() -> (w308:i32)
                n267 = property on="Test list" class="LstBox (strict)"() -> ("Item Names"=w309:string[])  [unwired: 2 in, 2 out]
                n268 = Index Array(array=w304, index=w305) -> (element=w306:string)
                n269 = Index Array(array=w309, index=w308) -> (element=w307:string)
                n270 = local write "State name"(w306) -> ()
                n271 = local write "Test name"(w307) -> ()
              }
              event "Test name": Value Change {
                n272 = event-data() -> ()  [unwired: 1 in, 6 out]
                n273 = property on="Test list" class="LstBox (strict)"() -> ("Item Names"=w315:string[])  [unwired: 2 in, 2 out]
                n274 = local read "Test list"() -> (w314:i32)
                n275 = Replace Array Subset(array=w315, new element="Test name", index=w314) -> (w312:string[])
                n276 = property on="Test list" class="LstBox (strict)"("Item Names"=w312) -> ()  [unwired: 2 in, 2 out]
              }
              event "State name": Value Change {
                n277 = event-data() -> ()  [unwired: 1 in, 6 out]
                n278 = local read "Influent list"() -> (w321:i32)
                n279 = property on="Influent list" class="LstBox (strict)"() -> ("Item Names"=w318:string[])  [unwired: 2 in, 2 out]
                n280 = local read "State Settings"() -> (w320:T3[][])
                n281 = Replace Array Subset(array=w318, new element="State name", index=w321) -> (w317:string[])
                n282 = property on="Influent list" class="LstBox (strict)"("Item Names"=w317) -> ()  [unwired: 2 in, 2 out]
                n283 = call "state name updater.vi"("State Names"=w317, "State Settings in"=w320) -> ("State Settings out"=w319:T3[][])
                n284 = local write "State Settings"(w319) -> ()
              }
            }
            "update gui" <- w160
          }
        }
      }
    }
  }
